vi "Split File.vi"(8 "error in (no error)":errorcluster, 11 "Data Logger Module in":refnum<class "Data Logger DBL Module.lvclass">) -> (0 "error out":errorcluster, 3 "Data Logger Module out":refnum<class "Data Logger DBL Module.lvclass">)   [LabVIEW 2020, in "VolatusData.lvlib" / "Data Logger DBL Module.lvclass"]
uses:
  Data Logger DBL Module.lvclass
  Data Logger DBL Module.lvclass/Data Logger DBL Module.ctl
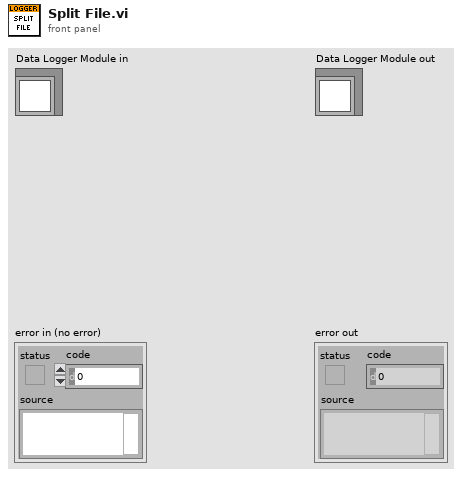
[diagram p1: front panel]
types:
  T1 = enum16{"open", "open or create", "create or replace", "create", "open (read-only)"}
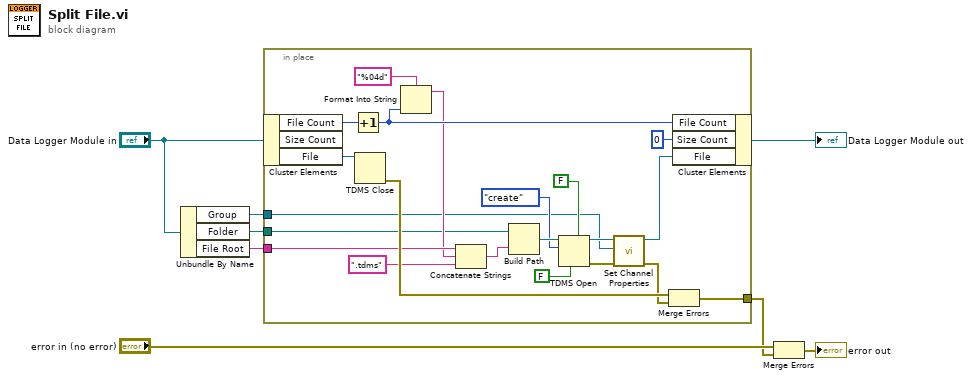
[diagram p0: block diagram]
diagram:
  n1 = Unbundle By Name("Data Logger Module in") -> ("Group"=w4:refnum<class "Group DBL.lvclass">, "Folder"=w5:path, "File Root"=w6:string)
  n2 = in-place {
    in-place-border: w6 -> [w24]
    in-place-border: w5 -> [w22]
    in-place-border: w4 -> [w13]
    in-place-border: [w10] -> w1
    n3 = in-place-cluster #1("Data Logger Module in") -> ("File Count"=w27:i32, "File"=w28:refnum<k34>)  [unwired: 1 out]
    n4 = Increment(x=w27) -> (x+1=w25:i32)
    n5 = TDMS Close(11:w28) -> (0:w29:errorcluster)  [unwired: 1 in, 1 out]
    n6 = Format Into String(format string="%04d", w25) -> (resulting string=w23:string)  [unwired: 2 in, 1 out]
    n7 = Concatenate Strings(w24, w23, ".tdms" ("string")) -> (w21:string)
    n8 = Build Path(base path=w22, name or relative path=w21) -> (appended path=w20:path)
    n9 = TDMS Open(5:FALSE ("create index file? (T)"), 6:FALSE ("disable buffering? (T)"), 10:T1."create" ("operation (0:open)"), 11:w20) -> (0:w14:errorcluster, 3:w15:refnum<k34>)  [unwired: 3 in]
    n10 = call "Set Channel Properties.vi"("error in (no error)"=w14, "Group"=w13, "File in"=w15) -> ("error out"=w12:errorcluster, "File"=w11:refnum<k34>)  [unwired: 5 in, 2 out]
    n11 = Merge Errors(w29, w12) -> (w10:errorcluster)
    n12 = in-place-cluster #1("File Count"=w25, "Size Count"=0, "File"=w11) -> (→"Data Logger Module out":refnum<class "Data Logger DBL Module.lvclass">)
  }
  n13 = Merge Errors("error in (no error)", w1) -> (→"error out":errorcluster)
